vi "AddModule_Item_OnCommand.vi"(10 "Command ID":string, 11 "Object":T1) -> ()   [LabVIEW 2012]
doc: "OnCommand\n\n\nInputs:\n---------------------\n- Command ID : String; \n- Object : U64; \n\nOutputs:\n---------------------\n\n\n----------------------------------------------\n6/8/2018 jcm\nZühlke Engineering AG\nCH-8952 Schlieren\nwww.zuehlke.com"
uses:
  <resource>/Framework/Providers/API/ItemRef.ctl
panel:
  out "error out":errorcluster
  in  "error in":errorcluster
  # "Connector Pane"
  # "Locals"
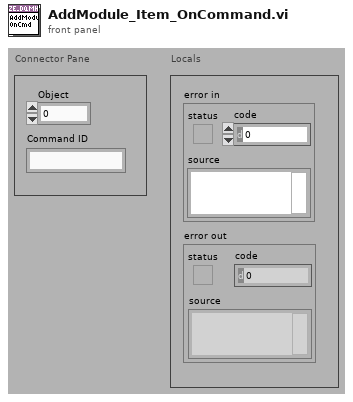
[diagram p1: front panel]
types:
  T1 = typedef "ItemRef.ctl" = u64
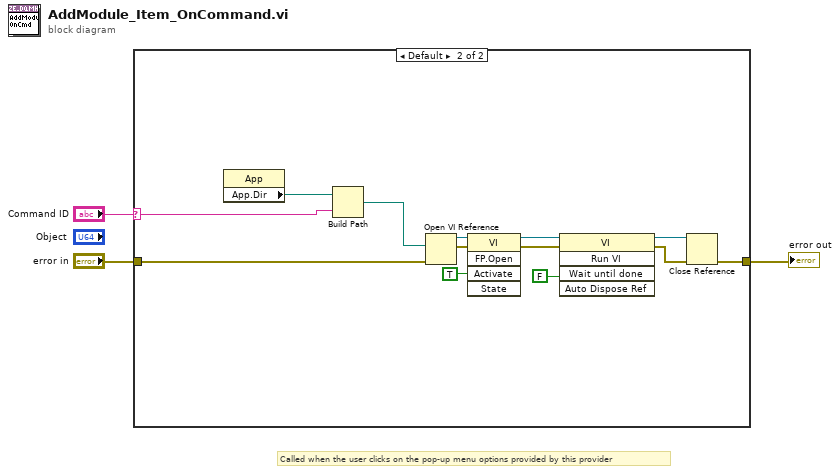
[diagram p0: block diagram]
diagram:
  # "Called when the user clicks on the pop-up menu options provided by this provider"
  n1 = case shown="Default" "Command ID" {
    selector: "Command ID" -> [_ w5]
    tunnel: "error in" -> [w4 w10]
    tunnel: [w4 w9] -> w1
    frame "" {
    }
    frame Default {
      n2 = property class="App"() -> ("App.Dir"=w7:path)  [unwired: 2 in, 2 out]
      n3 = Build Path(base path=w7, name or relative path=w5) -> (appended path=w6:path)
      n4 = Open VI Reference(vi path=w6, error in (no error)=w10) -> (vi reference=w12:refnum<vi>, error out=w13:errorcluster)  [unwired: 4 in]
      n5 = invoke class="VI" method="FP.Open"(reference=w12, error in=w13, "Activate"=TRUE ("Activate?")) -> (reference out=w14:refnum<vi>, error out=w15:errorcluster)  [unwired: 2 in, 3 out]
      n6 = invoke class="VI" method="Run VI"(reference=w14, error in=w15, "Wait until done"=FALSE ("Wait Until Done")) -> (reference out=w16:refnum<vi>, error out=w17:errorcluster)  [unwired: 2 in, 3 out]
      n7 = Close Reference(reference=w16, error in (no error)=w17) -> (error out=w9:errorcluster)
    }
  }
  "error out" <- w1
